vi "Dashboard Main_Fixed_1280x768.vi"() -> ()   [LabVIEW 2023]
uses:
  <vilib>/event_ctls.llb/eventvkey.ctl
  <vilib>/Rock Robotics/Network Tables/NT Read Numeric Array.vi
  <vilib>/Rock Robotics/Network Tables/NT Read Boolean.vi
  <vilib>/Rock Robotics/WPI/Dashboard/WPI_DashboardLogging Global.vi
panel:
  in  "Camera Settings Right":T1={"Frame Rate"=30, "Compression"=30, "Size"=1, "DB Camera Config"=FALSE} {"Frame Rate" scale=1.0..30.0; "Compression" scale=100.0..-1.0; "Size" items=["640x480", "320x240", "160x120"]}
  in  "Camera Name Right":string(combo)="No Camera Selection"
  out "Camera Perf":string
  in  "Camera Settings":T1={"Frame Rate"=30, "Compression"=30, "Size"=1, "DB Camera Config"=FALSE} {"Frame Rate" scale=1.0..30.0; "Compression" scale=100.0..-1.0; "Size" items=["640x480", "320x240", "160x120"]}
  in  "TCP":refnum<k5>
  in  "Rec Mode":enum32{"Stop", "Record", "Playback"}(radio)
  out "Robot IP":string
  out "Image Message":string="Timeout in Camera Communications"
  in  "Dashboard Tab":T2(tab)
  in  "Select Auto":string(combo)="Select Autonomous ..."
  out "NT Connection":bool
  out "MotorChart R":cluster{"Numeric":dbl, "Numeric":dbl}(graph)
  out "MotorChart L":cluster{"Numeric":dbl, "Numeric":dbl}(graph)
  out "MotorSliders R":cluster{"MotorSlide1":dbl, "MotorSlide2":dbl} {"MotorSlide2" scale=-1.0..1.0 scale format="%#_2e"; "MotorSlide1" scale=-1.0..1.0 scale format="%#_2e"}
  out "MotorSliders L":cluster{"MotorSlide1":dbl, "MotorSlide2":dbl} {"MotorSlide2" scale=-1.0..1.0 scale format="%#_2e"; "MotorSlide1" scale=-1.0..1.0 scale format="%#_2e"}
  out "Gyro":dbl(knob) scale=0.0..360.0
  out "JS1 Z":dbl(slide) scale=-1.0..1.0 scale format="%#_2e"
  out "JS1 Graph":cluster{"X":dbl, "Y":dbl}[](graph)
  out "JS1 Buttons":T3
  out "JS2 Z":dbl(slide) scale=-1.0..1.0 scale format="%#_2e"
  out "JS2 Graph":cluster{"X":dbl, "Y":dbl}[](graph)
  out "JS2 Buttons":T3
  out "Mode":T4(ring)=enum."Auto Disabled"
  out "Right Camera Perf":cluster{"Bandwidth (Mbps)":dbl, "FPS":dbl}
  out "Camera Image Right":T5(plugin-control)
  out "State":string
  out "Misaligned":bool
  out "Have Note":bool
  out "Box Ready":bool
  out "Arm on Target":bool
  out "Velocity Deg/Sec":dbl format="%11.1f"
  out "CO":dbl format="%11.2f"
  out "PV Deg":dbl format="%11.1f"
  out "SP Deg":dbl format="%11.1f"
  out "Lower Limit Switch":bool
  out "Arm Chart":T6(graph)
  out "Amp":bool
  out "Arm Blocked":bool
  out "Position":dbl
  out "Demand":dbl
  out "Error":dbl
  out "On Target":bool
  out "Floor":bool
  out "Shoot":bool
  out "Upright":bool
  out "Source":bool
  out "Right Vel":dbl format="%11.1f"
  out "Left Vel":dbl format="%11.1f"
  out "Right On Targ":bool
  out "Left On Targ":bool
  out "Right Upper (Virtual) Limit":bool
  out "Left Upper (Virtual) Limit":bool
  out "Right Low Limit":bool
  out "Right Co":dbl format="%11.2f"
  out "Right PV":dbl format="%11.1f"
  out "Left Co":dbl format="%11.2f"
  out "Left PV":dbl format="%11.1f"
  out "SP Inches":dbl format="%11.1f"
  out "Left Low Limit":bool
  out "Climb Chart":T7(graph)
  out "Left Pos":dbl
  out "Right Pos":dbl
  out "Dmd 2":dbl
  out "Right\nPosition":u8(slide) scale=0.0..100.0
  out "Left\nPosition":u8(slide) scale=0.0..100.0
  out "Dmd":u8(slide) scale=0.0..100.0
  out "Climb Blocked":bool
  out "Selected":string
  out "Step":string
  out "Error Dist":dbl
  in  "Test Slider":dbl(slide) scale=0.0..100.0 scale format="%#_3g"
  in  "On/Off":bool caption="Solenoid"
  in  "Test Name":u16(ring) items=["Select the test to run..."]
  in  "Test Tree":string(tree)
  in  "Motor":cluster{"Value":dbl, "Enable":bool} {"Value" scale=-1.0..1.0 scale format="%#_3g"}
  out "Progress":T8 {"Test Progress" scale=0.0..100.0}
  in  "Rev/Fwd":cluster{"Forward":bool, "Reverse":bool}
  in  "Test Ring":u16(ring) items=["Monochrome", "Color"]
  in  "CheckList":i32(listbox)
  out "Tree":string(tree)
  out "Camera Image":T5(plugin-control)
  out "Background":bool
  in  "Camera Name":string(combo)="No Camera Selection"
  # "HW"
  # "HW"
  # "Joysticks"
  # "Drive Motors"
  # "Front"
  # "Right"
  # "Left"
  # "Back"
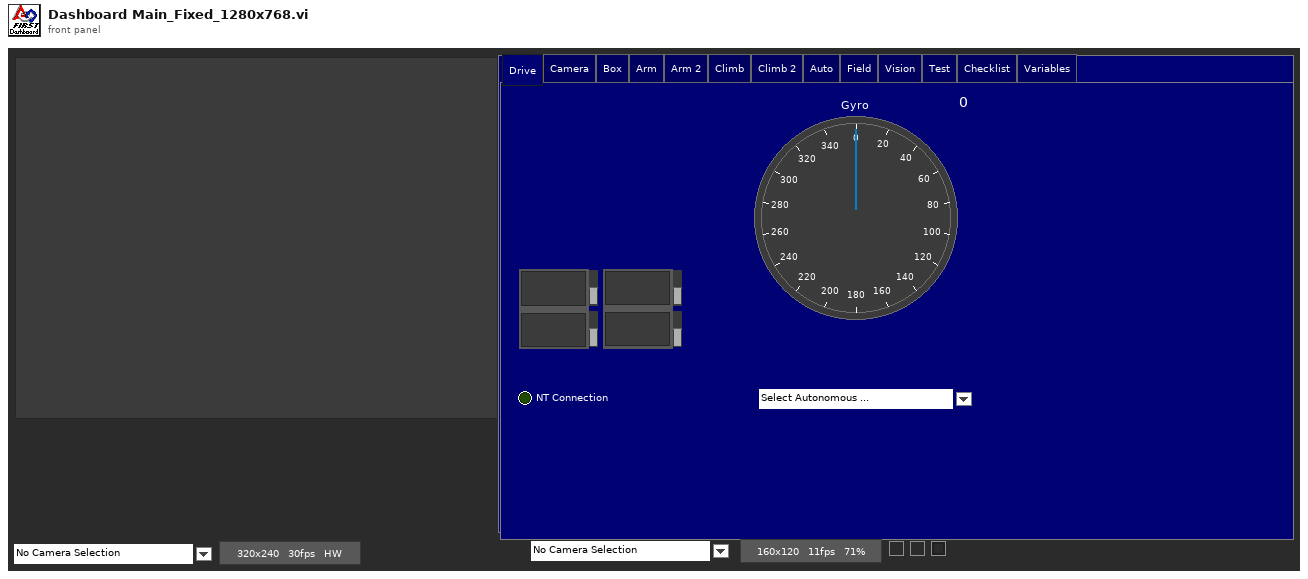
[diagram p1: front panel]
types:
  T1 = cluster{"Frame Rate":i32, "Compression":i32, "Size":u16, "DB Camera Config":bool}
  T2 = enum32{"Drive", "Camera", "Box", "Arm", "Arm 2", "Climb", "Climb 2", "Auto", "Field", "Vision", "Test", "Checklist", "Variables"}
  T3 = cluster{bool, bool, bool, bool, bool, bool, bool, bool, bool, bool, bool, bool}
  T4 = enum8{"Tele-Op Disabled", "Tele-Op Enabled", "Auto Disabled", "Auto Enabled", "Test Disabled", "Test Enabled", "Disconnected", "No Code", "E-Stop"}
  T5 = typedef "IMAQ Image.ctl" = refnum<image>
  T6 = cluster{"value":dbl, "value":dbl, "value":dbl, "value":dbl}
  T7 = cluster{"value":dbl, "value":dbl, "value":dbl, "value":dbl, "value":dbl}
  T8 = cluster{"Test Progress":u8, "Test Progress Text":string}
  T9 = cluster{"Save Path":path, "Interval (s)":dbl, "Keep":i32}
  T10 = enum32{"Drive", "Camera", "Basic", "Custom", "Test", "Commands", "Checklist", "Variables"}
  T11 = typedef "Image Type" = u32
  T12 = cluster{"Error Strings":string, "Disable Counts":cluster{u16, u16}, "Rail Faults":cluster{u16, u16, u16}, "Robot IP":string, "DB Mode":u8, "Event Info":cluster{"Name":string, "Type":u8, "Number":u16, "Replay":u8}}
  T13 = cluster{"Storage":cluster{"Disk Free":u64, "RAM Block":u32, "RAM free":u32}, "CPU Utilization":cluster{"CPU % ISR":sgl, "CPU % Time Crit":sgl, "CPU % Timed Str":sgl, "CPU % High":sgl, "CPU % Above":sgl, "CPU % Normal":sgl, "CPU % Low":sgl}, "CAN":cluster{"% Bus Utilization":sgl, "Bus Off Cnt":u32, "TX_FIFO Full Cnt":u32, "Receive Error Cnt":u8, "Transmit Error Cnt":u8}, "HID":cluster{"HID Outputs":u32, "Rumble Low":u16, "Rumble High":u16}[]}
  T14 = cluster{"Status bits":cluster{"Test Mode":bool, "Autonomous":bool, "Enabled":bool, "Code Start":bool, "Brownout":bool, "Reserved 2":bool, "Reserved 3":bool, "E-Stop":bool}, "Code Trace":cluster{"Disabled":bool, "TeleOp":bool, "Auto":bool, "Test":bool}, "Controller Type":enum16{"unknown", "cRIO", "roboRio"}, "Code?":enum16{"unknown", "noCode", "code"}, "Battery V":dbl}
  T15 = cluster{"Control Bits":cluster{"TestMode":bool, "Autonomous":bool, "Enabled":bool, "FMS Present":bool, bool, bool, bool, "E-Stop":bool}, "Team Station ":u8, "Countdown":sgl, "Joystick Values":cluster{"Axes":dbl[], "Buttons":bool[], "POVs":i16[]}[]}
  T16 = cluster{"Axes":dbl[], "Buttons":bool[], "POVs":i16[]}[]
  T17 = cluster{"Axes":dbl[], "Buttons":bool[], "POVs":i16[]}
  T18 = cluster{"Buttons[0]":bool, "Buttons[1]":bool, "Buttons[2]":bool, "Buttons[3]":bool, "Buttons[4]":bool, "Buttons[5]":bool, "Buttons[6]":bool, "Buttons[7]":bool, "Buttons[8]":bool, "Buttons[9]":bool, "Buttons[10]":bool, "Buttons[11]":bool}
  T19 = cluster{"Camera Image":refnum<vi>, "Dashboard Tab":refnum<vi>, "Background":refnum<vi>, "Rec Mode":refnum<vi>, "Test Slider":refnum<vi>, "On/Off ":refnum<vi>, "Test Ring":refnum<vi>, "Rev/Fwd":refnum<vi>, "Test Name":refnum<vi>, "Motor":refnum<vi>, "Progress":refnum<vi>, "CheckList":refnum<vi>, "Tree":refnum<vi>, "Test Tree":refnum<vi>, "Camera Settings":refnum<vi>, "Camera Name":refnum<vi>, "Camera Perf":refnum<vi>, "Camera Settings Right":refnum<vi>, "Camera Name Right":refnum<vi>, "Camera Image Right":refnum<vi>}
  T20 = cluster{"Global Rectangle":i32[], "Contours":cluster{"Contour Type":u32, "ROI Type":u32, "Points":i32[]}[]}
  T21 = cluster{"Camera Name":string, string, "Saved DB Images Info":cluster{"Save Path":path, "Interval (s)":dbl, "Keep":i32}}
  T22 = cluster{"Camera Name Right":string, string, "Saved DB Images Info":cluster{"Save Path":path, "Interval (s)":dbl, "Keep":i32}}
  T23 = cluster{"Operation":enum16{"Update", "Clear"}, "Color Box":u32}[]
  T24 = typedef "eventvkey.ctl" = enum16{"ASCII", "Enter", "Return", "Shift", "Ctrl", "Alt", "Cmd", "Opt", "Caps", "NumLock", "Clear", "Break", "Up", "Down", "Left", "Right", "Insert", "Delete", "Home", "End", "PageUp", "PageDown", "Escape", "Help", "Pause", "ScrollLock", "F1", "F2", "F3", "F4", "F5", "F6", "F7", "F8", "F9", "F10", "F11", "F12", "F13", "F14", "F15", "F16", "F17", "F18", "F19", "F20", "F21", "F22", "F23", "F24", "Play", "VolumeUp", "VolumeDown", "Mute", "Two Byte Char"}
  T25 = cluster{"Image Size":bool, "Image Type":bool, "Pixel Value":bool, "ROI Information":bool, "Zoom Factor":bool}
  T26 = cluster{"Operation":enum16{"Update", "Clear"}, "Color Box":u32}
  T27 = cluster{"Shift":bool, "Ctrl":bool, "Alt":bool, "Cmd":bool, "Opt":bool}
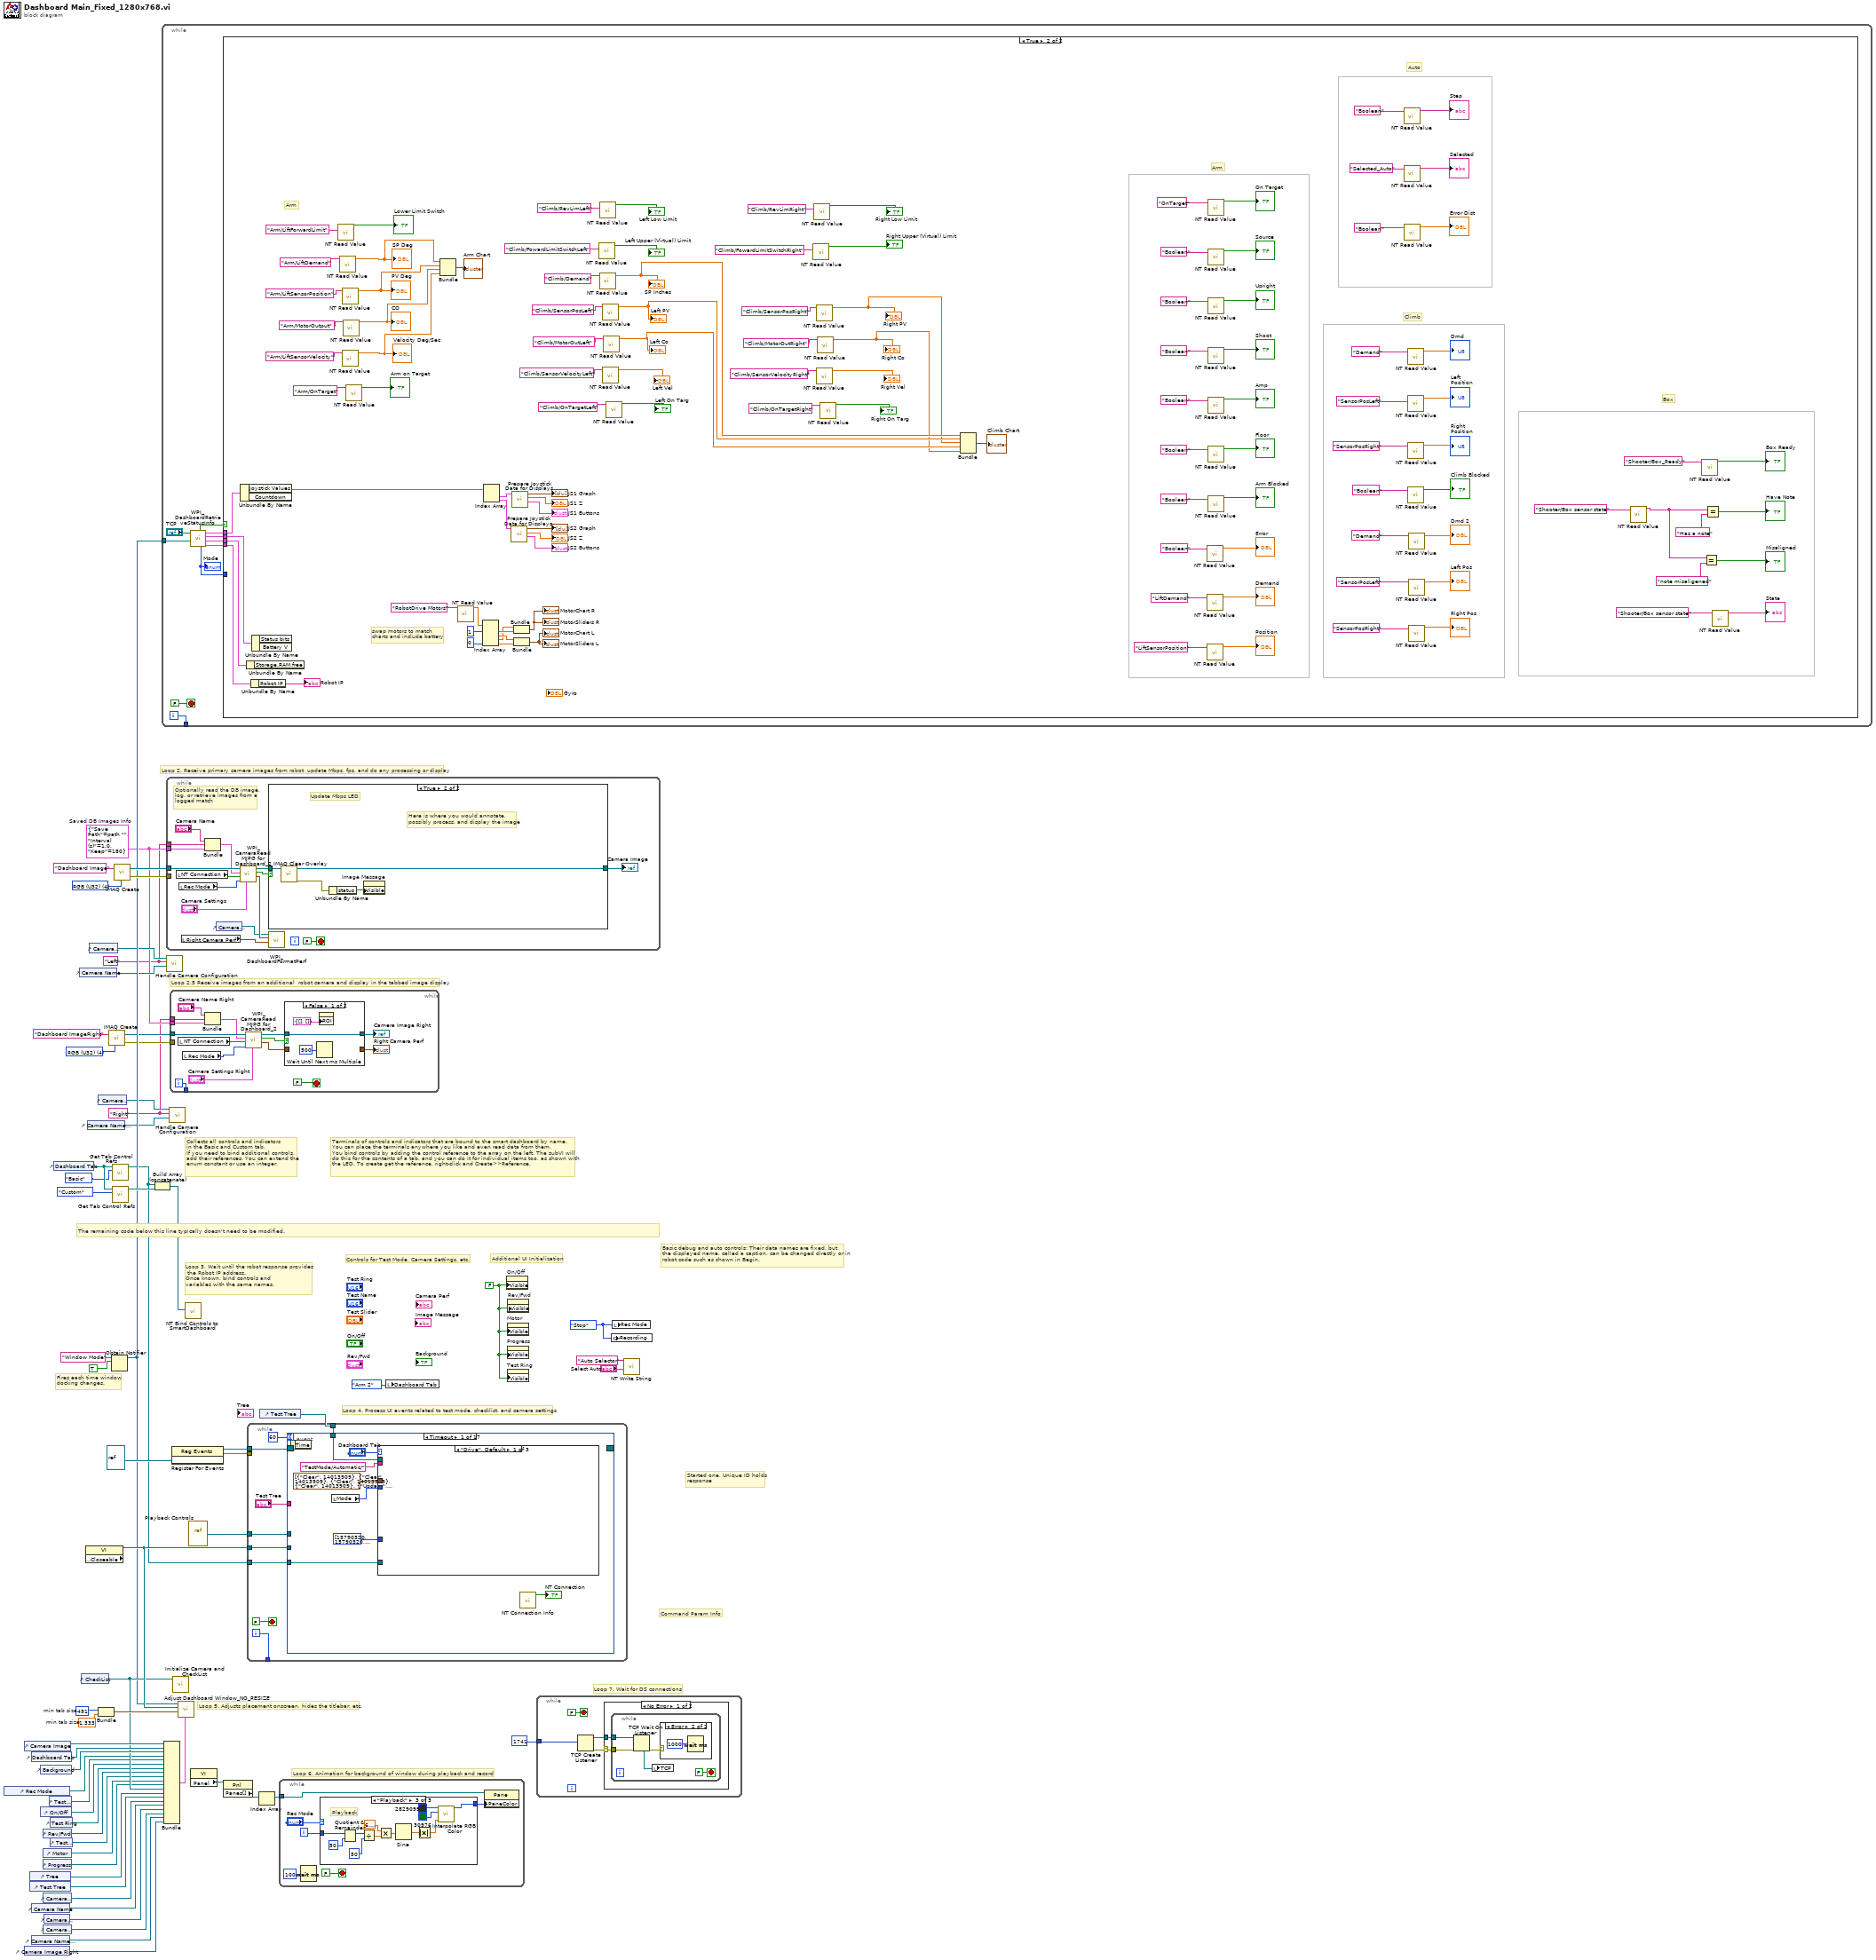
[diagram p0: block diagram]
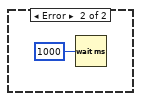
[diagram p4: hidden frame]
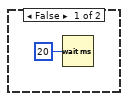
[diagram p5: hidden frame]
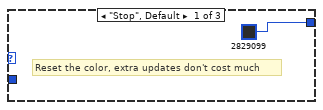
[diagram p6: hidden frame]
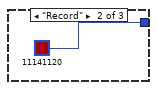
[diagram p7: hidden frame]
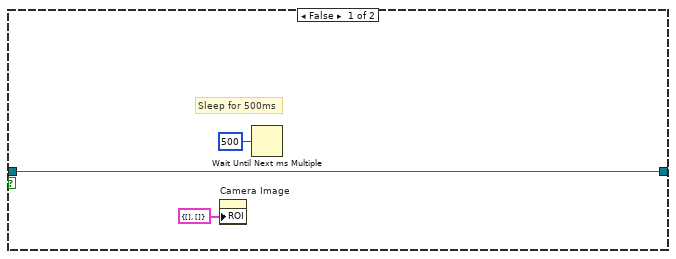
[diagram p8: hidden frame]
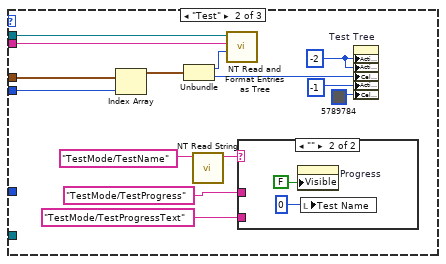
[diagram p9: hidden frame]
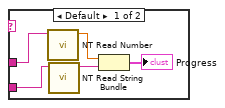
[diagram p10: hidden frame]
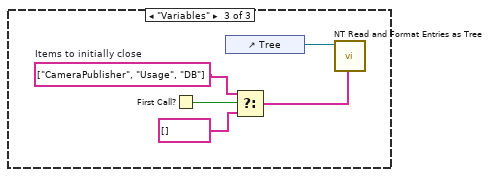
[diagram p11: hidden frame]
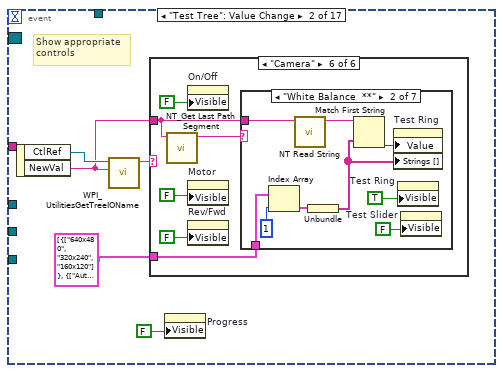
[diagram p12: hidden frame]
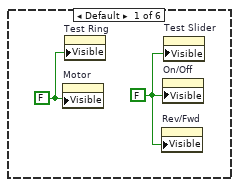
[diagram p13: hidden frame]
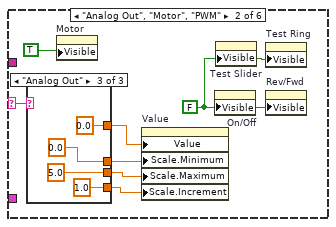
[diagram p14: hidden frame]
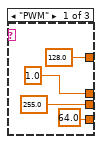
[diagram p15: hidden frame]
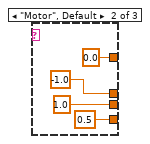
[diagram p16: hidden frame]
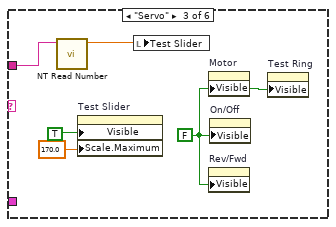
[diagram p17: hidden frame]
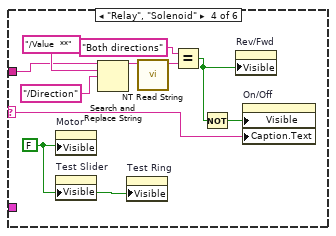
[diagram p18: hidden frame]
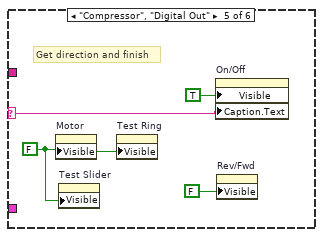
[diagram p19: hidden frame]
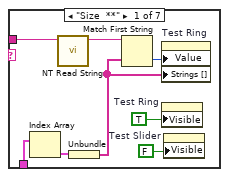
[diagram p20: hidden frame]
diagram:
  w4 = T9 {"Save Path"=path "", "Interval (s)"=1.0, "Keep"=180}  # Saved DB Images Info
  w3 = "Right"
  w2 = "Left"
  w14 = T11 4 items=["Grayscale (U8)", "Grayscale (I16)", "Grayscale (SGL)", "Complex (CSG)", "RGB (U32)", "HSL (U32)", "RGB (U64)"] ("Image Type")
  w42 = 491  # min tab size
  w41 = 1.333  # min tab size
  w49 = enum32{"Stop", "Record", "Playback"}."Stop" ("Rec Mode")
  w26 = FALSE ("Visible")
  w63 = T11 4 items=["Grayscale (U8)", "Grayscale (I16)", "Grayscale (SGL)", "Complex (CSG)", "RGB (U32)", "HSL (U32)", "RGB (U64)"] ("Image Type")
  # "Loop 2.5 Receive images from an additional  robot camera and display in the tabbed image display"
  # "Command Param Info"
  # "Started one, Unique ID holds\nresponse"
  # "Loop 7. Wait for DS connections"
  # "Basic debug and auto controls: Their data names are fixed, but\nthe displayed name, called a caption, can be changed directly or in\nrobot code such as shown in Begin."
  # "Controls for Test Mode, Camera Settings, etc."
  # "Additional UI Initialization"
  # "Loop 6. Animation for background of window during playback and record"
  # "Fires each time window\ndocking changes."
  # "Collects all controls and indicators\nin the Basic and Custom tab.\nIf you need to bind additional controls,\nadd their references. You can extend the\nenum constant or use an integer."
  # "The remaining code below this line typically doesn't need to be modified."
  # "Loop 4. Process UI events related to test mode, checklist, and camera settings"
  # "Terminals of controls and indicators that are bound to the smart dashboard by name.\nYou can place the terminals anywhere you like and even read data from them.\nYou bind controls by adding the control reference to the array on the left. The subVI will\ndo this for the contents of a tab, and you can do it for individual items too, as shown with\nthe LED. To create get the reference, right-click and Create>>Reference."
  # "Loop 3. Wait until the robot response provides\n the Robot IP address.\nOnce known, bind controls and\nvariables with the same names."
  # "Loop 5. Adjusts placement onscreen, hides the titlebar, etc."
  # "Loop 2. Receive primary camera images from robot, update Mbps, fps, and do any processing or display"
  n1 = control-ref of="Rec Mode"() -> (w32:refnum<vi>)
  n2 = control-ref of="Camera Image Right"() -> (w7:refnum<vi>)
  n3 = control-ref of="Camera Image"() -> (w44:refnum<vi>)
  n4 = control-ref of="Tree"() -> (w36:refnum<vi>)
  n5 = control-ref of="Test Tree"() -> (w35:refnum<vi>)
  n6 = control-ref of="Dashboard Tab"() -> (w43:refnum<vi>)
  n7 = control-ref of="Camera Name"() -> (w20:refnum<vi>)
  n8 = control-ref of="Camera Name Right"() -> (w8:refnum<vi>)
  n9 = control-ref of="Background"() -> (w39:refnum<vi>)
  n10 = control-ref of="On/Off"() -> (w30:refnum<vi>)
  n11 = control-ref of="Progress"() -> (w27:refnum<vi>)
  n12 = control-ref of="Camera Settings"() -> (w21:refnum<vi>)
  n13 = control-ref of="Camera Settings Right"() -> (w9:refnum<vi>)
  n14 = control-ref of="Rev/Fwd"() -> (w28:refnum<vi>)
  n15 = control-ref of="Motor"() -> (w33:refnum<vi>)
  n16 = control-ref of="Camera Perf"() -> (w19:refnum<vi>)
  n17 = control-ref of="Test Slider"() -> (w31:refnum<vi>)
  n18 = control-ref of="Test Ring"() -> (w29:refnum<vi>)
  n19 = control-ref of="Test Name"() -> (w34:refnum<vi>)
  n20 = control-ref of="Dashboard Tab"() -> (w47:refnum<vi>)
  n21 = control-ref of="Camera Name"() -> (w22:refnum<vi>)
  n22 = control-ref of="CheckList"() -> (w37:refnum<vi>)
  n23 = property class="VI" props=["Front Panel.Closeable"]() -> (reference out=w48:refnum<vi>)  [unwired: 2 in, 2 out]
  n24 = control-ref of="Camera Name Right"() -> (w10:refnum<vi>)
  n25 = control-ref of="Camera Settings"() -> (w23:refnum<vi>)
  n26 = control-ref of="Camera Settings Right"() -> (w11:refnum<vi>)
  n27 = Bundle("min tab size"=w42, "min tab size"=w41) -> (w40:cluster{"min tab size":i32, "min tab size":dbl})  [unwired: 1 in]
  n28 = call "IMAQ Create"("Image Name"="Dashboard ImageRight", "Image Type"=w14) -> ("New Image"=w13:T5, "error out"=w12:errorcluster)  [unwired: 2 in, 1 out]
  n29 = Obtain Notifier(name (unnamed)="Window Mode", notification data type=TRUE) -> (notifier out=w25:refnum<notifier>)  [unwired: 2 in, 2 out]
  n30 = call <vilib>:"Get Tab Control Refs.vi"("Page Index"=T10."Basic" ("Dashboard Tab"), "TabControl in"=w47) -> ("ControlsOnPage"=w18:refnum<vi>[])  [unwired: 9 in]
  n31 = call <vilib>:"Get Tab Control Refs.vi"("Page Index"=T10."Custom" ("Dashboard Tab"), "TabControl in"=w47) -> ("ControlsOnPage"=w46:refnum<vi>[])  [unwired: 9 in]
  n32 = call "IMAQ Create"("Image Name"="Dashboard Image", "Image Type"=w63) -> ("New Image"=w61:T5, "error out"=w60:errorcluster)  [unwired: 2 in, 1 out]
  n33 = Build Array (concatenate)(w18, w46) -> (w45:refnum<vi>[])
  n34 = while {
    tunnel: [w72] -> _
    tunnel: w25 -> [w64]
    i -> [w72]
    stop <- FALSE stop-if-true
    n35 = call <vilib>:"WPI_DashboardRetrieveStatusInfo.vi"("Window Mode Notifier"=w64, "TCP Cnx"="TCP") -> ("Power and Errors"=w67:T12, "Robot Metrics"=w70:T13, "Status Info"=w71:T14, "Control Info"=w68:T15, "Robot Mode"=w66:T4, "Process?"=w69:bool)  [unwired: 4 in]
    "Mode" <- w66
    n36 = case shown="True" w69 {
      tunnel: w71 -> [_ w188]
      tunnel: w70 -> [_ w187]
      tunnel: w68 -> [_ w186]
      tunnel: w67 -> [_ w185]
      tunnel: w66 -> [_ _]
      frame False {
        n37 = Wait (ms)(milliseconds to wait=u32 20) -> ()  [unwired: 1 out]
      }
      frame True {
        # "Auto"
        # "Climb"
        # "Arm"
        # "Box"
        # "Arm"
        # "swap motors to match\ncharts and include battery"
        n38 = Unbundle By Name(w186) -> ("Joystick Values"=w176:T16)  [unwired: 1 out]
        n39 = Unbundle By Name(w187) -> ()  [unwired: 1 out]
        n40 = Unbundle By Name(w185) -> ("Robot IP"=→"Robot IP":string)
        n41 = Unbundle By Name(w188) -> ()  [unwired: 2 out]
        n42 = call-poly <vilib>:"NT Read Value.vi"("name"="Arm/LiftForwardLimit") -> ("value"=→"Lower Limit Switch":bool)  [unwired: 8 in, 2 out]
        n43 = call-poly <vilib>:"NT Read Value.vi"("name"="Arm/LiftDemand") -> ("value"=w156:dbl)  [unwired: 8 in, 2 out]
        "SP Deg" <- w156
        n44 = call-poly <vilib>:"NT Read Value.vi"("name"="Arm/LiftSensorPosition") -> ("value"=w155:dbl)  [unwired: 8 in, 2 out]
        "PV Deg" <- w155
        n45 = call-poly <vilib>:"NT Read Value.vi"("name"="Arm/LiftSensorVelocity") -> ("value"=w153:dbl)  [unwired: 8 in, 2 out]
        "Velocity Deg/Sec" <- w153
        n46 = call-poly <vilib>:"NT Read Value.vi"("name"="Arm/MotorOutput") -> ("value"=w154:dbl)  [unwired: 8 in, 2 out]
        "CO" <- w154
        n47 = call-poly <vilib>:"NT Read Value.vi"("name"="Arm/OnTarget") -> ("value"=→"Arm on Target":bool)  [unwired: 8 in, 2 out]
        n48 = Bundle("value"=w156, "value"=w155, "value"=w154, "value"=w153) -> (→"Arm Chart":T6)  [unwired: 1 in]
        n49 = call-poly <vilib>:"NT Read Value.vi"("name"="RobotDrive Motors" ("Name")) -> ("value"=w166:dbl[])  [unwired: 8 in, 2 out]
        n50 = Index Array(array=w166, index #1=1, index #4=0) -> (element #1=w180:dbl, element #2=w181:dbl, element #3=w179:dbl, element #4=w184:dbl)  [unwired: 2 in]
        n51 = Index Array(array=w176) -> (element #1=w175:T17, element #2=w171:T17)  [unwired: 2 in]
        n52 = call "Prepare Joystick Data for Displays.vi"("Joystick Values"=w171) -> ("Buttons"=→"JS2 Buttons":T18, "Z Axis"=→"JS2 Z":dbl, "Cartesian Data"=→"JS2 Graph":cluster{"X axis":dbl, "X axis":dbl}[])  [unwired: 8 in]
        n53 = call "Prepare Joystick Data for Displays.vi"("Joystick Values"=w175) -> ("Buttons"=→"JS1 Buttons":T18, "Z Axis"=→"JS1 Z":dbl, "Cartesian Data"=→"JS1 Graph":cluster{"X axis":dbl, "X axis":dbl}[])  [unwired: 8 in]
        n54 = Bundle("Numeric"=w179, "Numeric"=w180) -> (→"MotorChart R" →"MotorSliders R":cluster{"Numeric":dbl, "Numeric":dbl})  [unwired: 1 in]
        n55 = Bundle("Numeric"=w181, "Numeric"=w184) -> (→"MotorChart L" →"MotorSliders L":cluster{"Numeric":dbl, "Numeric":dbl})  [unwired: 1 in]
        n56 = call-poly <vilib>:"NT Read Value.vi"("name"="Climb/FowardLimitSwitchLeft") -> ("value"=→"Left Upper (Virtual) Limit":bool)  [unwired: 8 in, 2 out]
        n57 = call-poly <vilib>:"NT Read Value.vi"("name"="Climb/Demand") -> ("value"=w129:dbl)  [unwired: 8 in, 2 out]
        "SP Inches" <- w129
        n58 = call-poly <vilib>:"NT Read Value.vi"("name"="Climb/RevLimLeft") -> ("value"=→"Left Low Limit":bool)  [unwired: 8 in, 2 out]
        n59 = call-poly <vilib>:"NT Read Value.vi"("name"="Climb/SensorPosLeft") -> ("value"=w128:dbl)  [unwired: 8 in, 2 out]
        "Left PV" <- w128
        n60 = call-poly <vilib>:"NT Read Value.vi"("name"="Climb/SensorVelocityLeft") -> ("value"=→"Left Vel":dbl)  [unwired: 8 in, 2 out]
        n61 = call-poly <vilib>:"NT Read Value.vi"("name"="Climb/MotorOutLeft") -> ("value"=w126:dbl)  [unwired: 8 in, 2 out]
        "Left Co" <- w126
        n62 = call-poly <vilib>:"NT Read Value.vi"("name"="Climb/OnTargetLeft") -> ("value"=→"Left On Targ":bool)  [unwired: 8 in, 2 out]
        n63 = call-poly <vilib>:"NT Read Value.vi"("name"="Climb/FowardLimitSwitchRight") -> ("value"=→"Right Upper (Virtual) Limit":bool)  [unwired: 8 in, 2 out]
        n64 = call-poly <vilib>:"NT Read Value.vi"("name"="Climb/RevLimRight") -> ("value"=→"Right Low Limit":bool)  [unwired: 8 in, 2 out]
        n65 = call-poly <vilib>:"NT Read Value.vi"("name"="Climb/SensorPosRight") -> ("value"=w127:dbl)  [unwired: 8 in, 2 out]
        "Right PV" <- w127
        n66 = call-poly <vilib>:"NT Read Value.vi"("name"="Climb/SensorVelocityRight") -> ("value"=→"Right Vel":dbl)  [unwired: 8 in, 2 out]
        n67 = call-poly <vilib>:"NT Read Value.vi"("name"="Climb/MotorOutRight") -> ("value"=w125:dbl)  [unwired: 8 in, 2 out]
        "Right Co" <- w125
        n68 = call-poly <vilib>:"NT Read Value.vi"("name"="Climb/OnTargetRight") -> ("value"=→"Right On Targ":bool)  [unwired: 8 in, 2 out]
        n69 = Bundle("value"=w129, "value"=w128, "value"=w127, "value"=w126, "value"=w125) -> (→"Climb Chart":T7)  [unwired: 1 in]
        n70 = call-poly <vilib>:"NT Read Value.vi"("name"="Boolean") -> ("value"=→"Error":dbl)  [unwired: 8 in, 2 out]
        n71 = call-poly <vilib>:"NT Read Value.vi"("name"="LiftDemand") -> ("value"=→"Demand":dbl)  [unwired: 8 in, 2 out]
        n72 = call-poly <vilib>:"NT Read Value.vi"("name"="LiftSensorPosition") -> ("value"=→"Position":dbl)  [unwired: 8 in, 2 out]
        n73 = call-poly <vilib>:"NT Read Value.vi"("name"="OnTarget") -> ("value"=→"On Target":bool)  [unwired: 8 in, 2 out]
        n74 = call-poly <vilib>:"NT Read Value.vi"("name"="Boolean") -> ("value"=→"Source":bool)  [unwired: 8 in, 2 out]
        n75 = call-poly <vilib>:"NT Read Value.vi"("name"="Boolean") -> ("value"=→"Upright":bool)  [unwired: 8 in, 2 out]
        n76 = call-poly <vilib>:"NT Read Value.vi"("name"="Boolean") -> ("value"=→"Shoot":bool)  [unwired: 8 in, 2 out]
        n77 = call-poly <vilib>:"NT Read Value.vi"("name"="Boolean") -> ("value"=→"Amp":bool)  [unwired: 8 in, 2 out]
        n78 = call-poly <vilib>:"NT Read Value.vi"("name"="Boolean") -> ("value"=→"Floor":bool)  [unwired: 8 in, 2 out]
        n79 = call-poly <vilib>:"NT Read Value.vi"("name"="Boolean") -> ("value"=→"Arm Blocked":bool)  [unwired: 8 in, 2 out]
        n80 = call-poly <vilib>:"NT Read Value.vi"("name"="Boolean") -> ("value"=→"Step":string)  [unwired: 8 in, 2 out]
        n81 = call-poly <vilib>:"NT Read Value.vi"("name"="Selected_Auto") -> ("value"=→"Selected":string)  [unwired: 8 in, 2 out]
        n82 = call-poly <vilib>:"NT Read Value.vi"("name"="Boolean") -> ("value"=→"Error Dist":dbl)  [unwired: 8 in, 2 out]
        n83 = call-poly <vilib>:"NT Read Value.vi"("name"="Demand") -> ("value"=→"Dmd":dbl)  [unwired: 8 in, 2 out]
        n84 = call-poly <vilib>:"NT Read Value.vi"("name"="SensorPosLeft") -> ("value"=→"Left\nPosition":dbl)  [unwired: 8 in, 2 out]
        n85 = call-poly <vilib>:"NT Read Value.vi"("name"="SensorPosRight") -> ("value"=→"Right\nPosition":dbl)  [unwired: 8 in, 2 out]
        n86 = call-poly <vilib>:"NT Read Value.vi"("name"="Boolean") -> ("value"=→"Climb Blocked":bool)  [unwired: 8 in, 2 out]
        n87 = call-poly <vilib>:"NT Read Value.vi"("name"="Demand") -> ("value"=→"Dmd 2":dbl)  [unwired: 8 in, 2 out]
        n88 = call-poly <vilib>:"NT Read Value.vi"("name"="SensorPosLeft") -> ("value"=→"Left Pos":dbl)  [unwired: 8 in, 2 out]
        n89 = call-poly <vilib>:"NT Read Value.vi"("name"="SensorPosRight") -> ("value"=→"Right Pos":dbl)  [unwired: 8 in, 2 out]
        n90 = call-poly <vilib>:"NT Read Value.vi"("name"="Shooter/Box sensor state") -> ("value"=w77:string)  [unwired: 8 in, 2 out]
        n91 = call-poly <vilib>:"NT Read Value.vi"("name"="Shooter/Box_Ready") -> ("value"=→"Box Ready":bool)  [unwired: 8 in, 2 out]
        n92 = Equal?(x=w77, y="note misaligened") -> (x = y?=→"Misaligned":bool)
        n93 = Equal?(x=w77, y="Has a note") -> (x = y?=→"Have Note":bool)
        n94 = call-poly <vilib>:"NT Read Value.vi"("name"="Shooter/Box sensor state") -> ("value"=→"State":string)  [unwired: 8 in, 2 out]
      }
    }
  }
  n95 = Bundle("Camera Image"=w44, "Dashboard Tab"=w43, "Background"=w39, "Rec Mode"=w32, "Test Slider"=w31, "On/Off"=w30, "Test Ring"=w29, "Rev/Fwd"=w28, "Test Name"=w34, "Motor"=w33, "Progress"=w27, "CheckList"=w37, "Tree"=w36, "Test Tree"=w35, "Camera Settings"=w21, "Camera Name"=w20, "Camera Perf"=w19, "Camera Settings Right"=w9, "Camera Name Right"=w8, "Camera Image Right"=w7) -> (w38:T19)  [unwired: 1 in]
  n96 = call "Handle Camera Configuration.vi"("CameraNameRef"=w22, "Display Name"=w2, "ClusterRef"=w23) -> ()  [unwired: 9 in]
  n97 = while {
    tunnel: w61 -> [w202]
    tunnel: w60 -> [_]
    tunnel: w4 -> [w195]
    tunnel: w2 -> [w192]
    stop <- FALSE stop-if-true
    # "Optionally read the DB image,\nlog, or retrieve images from a\nlogged match"
    n98 = local read "NT Connection"() -> (w196:bool)
    n99 = local read "Rec Mode"() -> (w199:enum32{"Stop", "Record", "Playback"})
    n100 = local read "Right Camera Perf"() -> (w190:cluster{"Bandwidth (Mbps)":dbl, "FPS":dbl})
    n101 = Bundle("Camera Name"="Camera Name", w192, "Saved DB Images Info"=w195) -> (w194:T21)  [unwired: 1 in]
    n102 = control-ref of="Camera Perf"() -> (w189:refnum<vi>)
    n103 = call <vilib>:"WPI_CameraRead MJPG for Dashboard_2.vi"("Camera Settings"="Camera Settings", "Rec Mode"=w199, "NT Connection"=w196, "Capture Info"=w194, "Image in"=w202) -> ("perf info"=w191:cluster{"Bandwidth (Mbps)":dbl, "fps":dbl}, "Active"=w200:bool, "Image\\ out"=w201:T5)  [unwired: 4 in]
    n104 = case shown="True" w200 {
      tunnel: w201 -> [w205 w208]
      tunnel: [w205 w207] -> w197
      frame False {
        # "Sleep for 500ms"
        n105 = property on="Camera Image" class="ImageControl"("ROI"=T20 {"Global Rectangle"=[], "Contours"=[]}) -> ()  [unwired: 2 in, 2 out]
        n106 = Wait Until Next ms Multiple(millisecond multiple=u32 500) -> ()  [unwired: 1 out]
      }
      frame True {
        # "Here is where you would annotate,\npossibly process, and display the image"
        # "Update Mbps LED"
        n107 = call "IMAQ Clear Overlay"("Image"=w208) -> ("error out"=w209:errorcluster, "Image Out"=w207:T5)  [unwired: 2 in, 7 out]
        n108 = Unbundle By Name(w209) -> ("status"=w210:bool)
        n109 = property on="Image Message" class="Str"("Visible"=w210) -> ()  [unwired: 2 in, 2 out]
      }
    }
    "Camera Image" <- w197
    n110 = call <vilib>:"WPI_DashboardFormatPerf.vi"("Right Camera Perf"=w190, "Performance"=w191, "String in"=w189) -> ()  [unwired: 9 in]
  }
  n111 = call "Handle Camera Configuration.vi"("CameraNameRef"=w10, "Display Name"=w3, "ClusterRef"=w11) -> ()  [unwired: 9 in]
  n112 = while {
    tunnel: w13 -> [w225]
    tunnel: w12 -> [_]
    tunnel: [w220] -> _
    tunnel: w4 -> [w216]
    tunnel: w3 -> [w213]
    i -> [w220]
    stop <- FALSE stop-if-true
    n113 = local read "NT Connection"() -> (w217:bool)
    n114 = local read "Rec Mode"() -> (w224:enum32{"Stop", "Record", "Playback"})
    n115 = Bundle("Camera Name Right"="Camera Name Right", w213, "Saved DB Images Info"=w216) -> (w215:T22)  [unwired: 1 in]
    n116 = call <vilib>:"WPI_CameraRead MJPG for Dashboard_2.vi"("Camera Settings"="Camera Settings Right", "Rec Mode"=w224, "NT Connection"=w217, "Capture Info"=w215, "Image in"=w225) -> ("perf info"=w211:cluster{"Bandwidth (Mbps)":dbl, "fps":dbl}, "Active"=w219:bool, "Image\\ out"=w222:T5)  [unwired: 4 in]
    n117 = case shown="False" w219 {
      tunnel: w222 -> [w227 w230]
      tunnel: [w227 w230] -> w218
      tunnel: [_ w229] -> w212
      tunnel: w211 -> [_ w229]
      frame False {
        n118 = Wait Until Next ms Multiple(millisecond multiple=u32 500) -> ()  [unwired: 1 out]
        n119 = property on="Camera Image Right" class="ImageControl"("ROI"=T20 {"Global Rectangle"=[], "Contours"=[]}) -> ()  [unwired: 2 in, 2 out]
      }
      frame True {
      }
    }
    "Camera Image Right" <- w218
    "Right Camera Perf" <- w212
  }
  n120 = register-events(refnum<vi> refnum) -> (reference out=w52:refnum<event-registration>, error out=w51:errorcluster)  [unwired: 2 in]
  n121 = call "Initialize Camera and CheckList.vi"("ListBox in"=w37) -> ()  [unwired: 11 in]
  n122 = call "Adjust Dashboard Window_NO_RESIZE.vi"("Sizing Refnums"=w38, "Size Constraints"=w40, "VI"=w48, "WIn Mode"=w25) -> ()  [unwired: 8 in]
  n123 = call <vilib>:"NT Bind Controls to SmartDashboard.vi"("Bound Control Refs"=w45) -> ()  [unwired: 11 in]
  n124 = vi-ref "Playback Controls.vi"() -> (w53:refnum<vi>)
  n125 = property class="VI"() -> ("Panel"=w55:refnum<vi>)  [unwired: 2 in, 2 out]
  n126 = property class="Pnl"(reference=w55) -> ("Panes[]"=w56:refnum<vi>[])  [unwired: 1 in, 2 out]
  n127 = Index Array(array=w56) -> (element=w54:refnum<vi>)  [unwired: 1 in]
  n128 = control-ref of="Test Tree"() -> (w57:refnum<vi>)
  n129 = while {
    tunnel: [w236] -> _
    tunnel: w57 -> [w235]
    tunnel: w53 -> [w234]
    tunnel: w52 -> [w233]
    tunnel: w51 -> [_]
    tunnel: w48 -> [w232]
    tunnel: w18 -> [w231]
    i -> [w236]
    stop <- FALSE stop-if-true
    n130 = event shown="[0] Timeout" {
      selector: w233 -> [_ _ _ _ _ _ _ _ _ _ _ _ _ _ _ _ _]
      dyn-events: [_ _ _ _ _ _ _ _ _ _ _ _ _ w440 _ _ _] -> _
      timeout: u32 60 ("milliseconds to wait") -> [_ _ _ _ _ _ _ _ _ _ _ _ _ _ _ _ _]
      tunnel: w235 -> [w246 _ _ _ _ _ _ _ _ _ _ _ _ _ _ _ _]
      tunnel: "Test Tree" -> [_ _ _ _ _ _ _ _ w413 w420 w421 w424 w431 _ _ _ _]
      tunnel: w234 -> [_ _ _ _ _ _ _ _ _ _ _ _ _ w442 _ w457 _]
      tunnel: w232 -> [_ _ _ _ _ _ _ _ _ _ _ _ _ w438 _ _ _]
      tunnel: w231 -> [w241 _ _ _ _ _ _ _ _ _ _ _ _ _ _ _ _]
      event Timeout {
        n131 = event-data() -> ()  [unwired: 1 in, 1 out]
        n132 = local read "Mode"() -> (w244:T4)
        n133 = case shown="\"Drive\", Default" "Dashboard Tab" {
          tunnel: w246 -> [_ w261 _]
          tunnel: "TestMode/Automatic/" ("Name Pattern") -> [_ w260 _]
          tunnel: T23 [{"Operation"=enum."Clear", "Color Box"=14013909}, {"Operation"=enum."Clear", "Color Box"=14013909}, {"Operation"=enum."Clear", "Color Box"=14013909}, {"Operation"=enum."Clear", "Color Box"=14013909}, {"Operation"=enum."Update", "Color Box"=14013909}, {"Operation"=enum."Update", "Color Box"=16777215}, {"Operation"=enum."Clear", "Color Box"=14013909}, {"Operation"=enum."Clear", "Color Box"=14013909}, {"Operation"=enum."Clear", "Color Box"=14013909}] -> [_ w253 _]
          tunnel: w244 -> [_ w252 _]
          tunnel: u32[] [15790320, 15790320, 15790320, 15790320, 16777215, 16777215, 15790320, 15790320, 15790320] -> [_ _ _]
          tunnel: w241 -> [_ _ _]
          frame "Drive", Default {
          }
          frame "Test" {
            w259 = -2 ("Active Item:Row Number")
            n134 = Index Array(array=w253, index=w252) -> (element=w254:T26)
            n135 = Unbundle(w254) -> ("Operation"=w255:enum16{"Update", "Clear"}, "Color Box"=w256:u32)
            n136 = call <vilib>:"NT Read String.vi"("name"="TestMode/TestName" ("Name")) -> ("value"=w250:string)  [unwired: 8 in, 2 out]
            n137 = call <vilib>:"NT Read and Format Entries as Tree.vi"("Operation"=w255, "Name Pattern"=w260, "Tree Refnum"=w261) -> ()  [unwired: 7 in, 2 out]
            n138 = case shown="\"\"" w250 {
              tunnel: "TestMode/TestProgress" ("Name") -> [w263 _]
              tunnel: "TestMode/TestProgressText" ("Name") -> [w262 _]
              frame Default {
                n139 = call <vilib>:"NT Read Number.vi"("name"=w263) -> ("value"=w264:dbl)  [unwired: 8 in, 2 out]
                n140 = call <vilib>:"NT Read String.vi"("name"=w262) -> ("value"=w265:string)  [unwired: 8 in, 2 out]
                n141 = Bundle("value"=w264, "value"=w265) -> (→"Progress":cluster{"value":dbl, "value":string})  [unwired: 1 in]
              }
              frame "" {
                n142 = property on="Progress" class="Clust (strict)"("Visible"=FALSE) -> ()  [unwired: 2 in, 2 out]
                n143 = local write "Test Name"(u16 0) -> ()
              }
            }
            n144 = property on="Test Tree" class="Tree (strict)"("Active Item Row Number"=w259, "ActiveColNum"=w259, "CellBG"=w256, "Active Item Row Number"=-1 ("Active Item:Row Number"), "CellBG"=u32 5789784 ("Color Box")) -> ()  [unwired: 2 in, 2 out]
          }
          frame "Variables" {
            w271 = string[] ["CameraPublisher", "Usage", "DB"]  # Items to initially close
            n145 = First Call?() -> (First Call?: T/F=w272:bool)
            n146 = control-ref of="Tree"() -> (w273:refnum<vi>)
            n147 = Select(t=w271, s=w272, f=string[] []) -> (s? t:f=w269:string[])
            n148 = call <vilib>:"NT Read and Format Entries as Tree.vi"("Tags to  Close"=w269, "Tree Refnum"=w273) -> ()  [unwired: 8 in, 2 out]
          }
        }
        n149 = call <vilib>:"NT Connection Info.vi"() -> ("Connected"=→"NT Connection":bool)  [unwired: 11 in]
      }
      event "Test Tree": Value Change {
        # "Show appropriate\ncontrols"
        n150 = event-data() -> ("CtlRef"=w277:refnum<vi>, "NewVal"=w275:string)  [unwired: 1 in]
        n151 = call <vilib>:"WPI_UtilitiesGetTreeIOName.vi"("NewVal"=w275, "TreeControl in"=w277) -> ("I/O Name"=w278:string)  [unwired: 9 in]
        n152 = case shown="\"Camera\"" w278 {
          selector: w278 -> [_ w285 _ w307 w316 _]
          tunnel: w275 -> [_ _ w304 w306 _ w323]
          tunnel: cluster{string[]}[] [{["640x480", "320x240", "160x120"]}, {["Auto", "Fixed indoor", "Fixed outdoor 1", "Fixed outdoor 2", "Fixed fluorescent 1", "Fixed fluorescent 2", "Hold current"]}, {["Auto", "Flicker-free 50 Hz", "Flicker-free 60 Hz", "Hold current"]}, {["None", "Prioritize frame rate", "Prioritize image quality"]}, {["Monochrome", "Color"]}] -> [_ _ _ _ _ w322]
          frame Default {
            w280 = FALSE ("Visible")
            w279 = FALSE ("Visible")
            n153 = property on="Motor" class="Clust (strict)"("Visible"=w279) -> ()  [unwired: 2 in, 2 out]
            n154 = property on="Test Ring" class="Ring (strict)"("Visible"=w279) -> ()  [unwired: 2 in, 2 out]
            n155 = property on="Rev/Fwd" class="Clust (strict)"("Visible"=w280) -> ()  [unwired: 2 in, 2 out]
            n156 = property on="On/Off" class="Bool (strict)"("Visible"=w280) -> ()  [unwired: 2 in, 2 out]
            n157 = property on="Test Slider" class="Slide (strict)"("Visible"=w280) -> ()  [unwired: 2 in, 2 out]
          }
          frame "Analog Out", "Motor", "PWM" {
            w286 = FALSE ("Visible")
            n158 = case shown="\"Analog Out\"" w285 {
              tunnel: [1.0 ("Value") -1.0 ("Value") 0.0 ("Value")] -> w284
              tunnel: [255.0 ("Value") 1.0 ("Value") 5.0 ("Value")] -> w283
              tunnel: [128.0 ("Value") 0.0 ("Value") 0.0 ("Value")] -> w282
              tunnel: [64.0 ("Value") 0.5 ("Value") 1.0 ("Value")] -> w281
              frame "PWM" {
              }
              frame "Motor", Default {
              }
              frame "Analog Out" {
              }
            }
            n159 = property on="Motor" class="Clust (strict)"("Visible"=TRUE) -> ()  [unwired: 2 in, 2 out]
            n160 = property on="Value" class="Slide (strict)"("Value"=w282, "Scale.Minimum"=w284, "Scale.Maximum"=w283, "Scale.Increment"=w281) -> ()  [unwired: 2 in, 2 out]
            n161 = property on="On/Off" class="Bool (strict)"("Visible"=w286) -> ()  [unwired: 2 in, 2 out]
            n162 = property on="Test Slider" class="Slide (strict)"("Visible"=w286) -> ()  [unwired: 2 in, 2 out]
            n163 = property on="Test Ring" class="Ring (strict)"("Visible"=w286) -> ()  [unwired: 2 in, 2 out]
            n164 = property on="Rev/Fwd" class="Clust (strict)"("Visible"=w286) -> ()  [unwired: 2 in, 2 out]
          }
          frame "Servo" {
            w302 = FALSE ("Visible")
            n165 = call <vilib>:"NT Read Number.vi"("name"=w304) -> ("value"=w303:dbl)  [unwired: 8 in, 2 out]
            n166 = property on="Test Slider" class="Slide (strict)"("Visible"=TRUE, "Scale.Maximum"=170.0 ("Scale.Range:Maximum")) -> ()  [unwired: 2 in, 2 out]
            n167 = local write "Test Slider"(w303) -> ()
            n168 = property on="Motor" class="Clust (strict)"("Visible"=w302) -> ()  [unwired: 2 in, 2 out]
            n169 = property on="Rev/Fwd" class="Clust (strict)"("Visible"=w302) -> ()  [unwired: 2 in, 2 out]
            n170 = property on="On/Off" class="Bool (strict)"("Visible"=w302) -> ()  [unwired: 2 in, 2 out]
            n171 = property on="Test Ring" class="Ring (strict)"("Visible"=w302) -> ()  [unwired: 2 in, 2 out]
          }
          frame "Relay", "Solenoid" {
            w305 = FALSE ("Visible")
            n172 = property on="Motor" class="Clust (strict)"("Visible"=w305) -> ()  [unwired: 2 in, 2 out]
            n173 = property on="Test Slider" class="Slide (strict)"("Visible"=w305) -> ()  [unwired: 2 in, 2 out]
            n174 = Search and Replace String(input string=w306, search string="/Value  **", replace string="/Direction") -> (result string=w312:string)  [unwired: 5 in, 3 out]
            n175 = property on="Test Ring" class="Ring (strict)"("Visible"=w305) -> ()  [unwired: 2 in, 2 out]
            n176 = call <vilib>:"NT Read String.vi"("name"=w312) -> ("value"=w310:string)  [unwired: 8 in, 2 out]
            n177 = Equal?(x="Both directions", y=w310) -> (x = y?=w308:bool)
            n178 = Not(x=w308) -> (.not. x?=w309:bool)
            n179 = property on="Rev/Fwd" class="Clust (strict)"("Visible"=w308) -> ()  [unwired: 2 in, 2 out]
            n180 = property on="On/Off" class="Bool (strict)"("Visible"=w309, "Caption.Text"=w307) -> ()  [unwired: 2 in, 2 out]
          }
          frame "Compressor", "Digital Out" {
            w315 = FALSE ("Visible")
            # "Get direction and finish"
            n181 = property on="Motor" class="Clust (strict)"("Visible"=w315) -> ()  [unwired: 2 in, 2 out]
            n182 = property on="Test Slider" class="Slide (strict)"("Visible"=w315) -> ()  [unwired: 2 in, 2 out]
            n183 = property on="Test Ring" class="Ring (strict)"("Visible"=w315) -> ()  [unwired: 2 in, 2 out]
            n184 = property on="On/Off" class="Bool (strict)"("Visible"=TRUE, "Caption.Text"=w316) -> ()  [unwired: 2 in, 2 out]
            n185 = property on="Rev/Fwd" class="Clust (strict)"("Visible"=FALSE) -> ()  [unwired: 2 in, 2 out]
          }
          frame "Camera" {
            n186 = call <vilib>:"NT_Get Last Path Segment.vi"("String in"=w323) -> ("String out"=w324:string)  [unwired: 10 in]
            n187 = property on="On/Off" class="Bool (strict)"("Visible"=FALSE) -> ()  [unwired: 2 in, 2 out]
            n188 = property on="Motor" class="Clust (strict)"("Visible"=FALSE) -> ()  [unwired: 2 in, 2 out]
            n189 = property on="Rev/Fwd" class="Clust (strict)"("Visible"=FALSE) -> ()  [unwired: 2 in, 2 out]
            n190 = case shown="\"White Balance  **\"" w324 {
              tunnel: w323 -> [w330 w339 w348 w357 w366 _ w372]
              tunnel: w322 -> [w328 w336 w345 w354 w363 _ _]
              frame "Size  **" {
                n191 = Index Array(array=w328) -> (element=w327:cluster{string[]})  [unwired: 1 in]
                n192 = call <vilib>:"NT Read String.vi"("name"=w330) -> ("value"=w329:string)  [unwired: 8 in, 2 out]
                n193 = Unbundle(w327) -> (w325:string[])
                n194 = Match First String(2:w325, 3:w329) -> (0:w326:i32)  [unwired: 1 out]
                n195 = property on="Test Ring" class="Ring (strict)"("Value"=w326, "Strings []"=w325) -> ()  [unwired: 2 in, 2 out]
                n196 = property on="Test Ring" class="Ring (strict)"("Visible"=TRUE) -> ()  [unwired: 2 in, 2 out]
                n197 = property on="Test Slider" class="Slide (strict)"("Visible"=FALSE) -> ()  [unwired: 2 in, 2 out]
              }
              frame "White Balance  **" {
                n198 = Index Array(array=w336, index=1) -> (element=w337:cluster{string[]})
                n199 = call <vilib>:"NT Read String.vi"("name"=w339) -> ("value"=w338:string)  [unwired: 8 in, 2 out]
                n200 = Unbundle(w337) -> (w334:string[])
                n201 = Match First String(2:w334, 3:w338) -> (0:w333:i32)  [unwired: 1 out]
                n202 = property on="Test Ring" class="Ring (strict)"("Value"=w333, "Strings []"=w334) -> ()  [unwired: 2 in, 2 out]
                n203 = property on="Test Ring" class="Ring (strict)"("Visible"=TRUE) -> ()  [unwired: 2 in, 2 out]
                n204 = property on="Test Slider" class="Slide (strict)"("Visible"=FALSE) -> ()  [unwired: 2 in, 2 out]
              }
              frame "Exposure  **" {
                n205 = Index Array(array=w345, index=2) -> (element=w346:cluster{string[]})
                n206 = call <vilib>:"NT Read String.vi"("name"=w348) -> ("value"=w347:string)  [unwired: 8 in, 2 out]
                n207 = Unbundle(w346) -> (w342:string[])
                n208 = Match First String(2:w342, 3:w347) -> (0:w343:i32)  [unwired: 1 out]
                n209 = property on="Test Ring" class="Ring (strict)"("Value"=w343, "Strings []"=w342) -> ()  [unwired: 2 in, 2 out]
                n210 = property on="Test Ring" class="Ring (strict)"("Visible"=TRUE) -> ()  [unwired: 2 in, 2 out]
                n211 = property on="Test Slider" class="Slide (strict)"("Visible"=FALSE) -> ()  [unwired: 2 in, 2 out]
              }
              frame "Exposure Priority  **" {
                n212 = Index Array(array=w354, index=3) -> (element=w355:cluster{string[]})
                n213 = call <vilib>:"NT Read String.vi"("name"=w357) -> ("value"=w356:string)  [unwired: 8 in, 2 out]
                n214 = Unbundle(w355) -> (w351:string[])
                n215 = Match First String(2:w351, 3:w356) -> (0:w352:i32)  [unwired: 1 out]
                n216 = property on="Test Ring" class="Ring (strict)"("Value"=w352, "Strings []"=w351) -> ()  [unwired: 2 in, 2 out]
                n217 = property on="Test Ring" class="Ring (strict)"("Visible"=TRUE) -> ()  [unwired: 2 in, 2 out]
                n218 = property on="Test Slider" class="Slide (strict)"("Visible"=FALSE) -> ()  [unwired: 2 in, 2 out]
              }
              frame "Color Enable  **" {
                n219 = Index Array(array=w363, index=4) -> (element=w364:cluster{string[]})
                n220 = call <vilib>:"NT Read String.vi"("name"=w366) -> ("value"=w365:string)  [unwired: 8 in, 2 out]
                n221 = Unbundle(w364) -> (w360:string[])
                n222 = Match First String(2:w360, 3:w365) -> (0:w361:i32)  [unwired: 1 out]
                n223 = property on="Test Ring" class="Ring (strict)"("Value"=w361, "Strings []"=w360) -> ()  [unwired: 2 in, 2 out]
                n224 = property on="Test Ring" class="Ring (strict)"("Visible"=TRUE) -> ()  [unwired: 2 in, 2 out]
                n225 = property on="Test Slider" class="Slide (strict)"("Visible"=FALSE) -> ()  [unwired: 2 in, 2 out]
              }
              frame Default {
                n226 = property on="Test Ring" class="Ring (strict)"("Visible"=FALSE) -> ()  [unwired: 2 in, 2 out]
                n227 = property on="Test Slider" class="Slide (strict)"("Visible"=FALSE) -> ()  [unwired: 2 in, 2 out]
              }
              frame "Brightness  **", "Color Level  **", "Compression  **", "FPS  **", "Sharpness  **" {
                n228 = call <vilib>:"NT Read Number.vi"("name"=w372) -> ("value"=w371:dbl)  [unwired: 8 in, 2 out]
                n229 = local write "Test Slider"(w371) -> ()
                n230 = property on="Test Ring" class="Ring (strict)"("Visible"=FALSE) -> ()  [unwired: 2 in, 2 out]
                n231 = property on="Test Slider" class="Slide (strict)"("Visible"=TRUE, "Scale.Maximum"=100.0 ("Scale.Range:Maximum")) -> ()  [unwired: 2 in, 2 out]
              }
            }
          }
        }
        n232 = property on="Progress" class="Clust (strict)"("Visible"=FALSE) -> ()  [unwired: 2 in, 2 out]
      }
      event "Test Name": Mouse Enter {
        # "Populate the ring with the list of tests"
        n233 = event-data() -> ()  [unwired: 1 in, 1 out]
        n234 = call <vilib>:"NT Read String Array.vi"("name"="TestMode/TestList" ("Name")) -> ("value"=w379:string[])  [unwired: 8 in, 2 out]
        n235 = Build Array (concatenate)("Select the test to run...", w379) -> (w378:string[])
        n236 = property on="Test Name" class="Ring (strict)"("Strings []"=w378) -> ()  [unwired: 2 in, 2 out]
      }
      event "Test Name": Value Change {
        w380 = FALSE ("Visible")
        # "Tell the robot the test name to run"
        n237 = event-data() -> ("NewVal"=w384:u16)  [unwired: 1 in]
        n238 = property on="Test Name" class="Ring (strict)"() -> ("Strings []"=w385:string[])  [unwired: 2 in, 2 out]
        n239 = local write "Progress"(T8 {"Test Progress"=0, "Test Progress Text"=""} ("Progress")) -> ()
        n240 = Index Array(array=w385, index=w384) -> (element=w383:string)
        n241 = call <vilib>:"NT Write String.vi"("value"=w383, "name"="TestMode/TestName" ("Name")) -> ()  [unwired: 9 in, 1 out]
        n242 = property on="Progress" class="Clust (strict)"("Visible"=TRUE) -> ()  [unwired: 2 in, 2 out]
        n243 = property on="Motor" class="Clust (strict)"("Visible"=w380) -> ()  [unwired: 2 in, 2 out]
        n244 = property on="Test Slider" class="Slide (strict)"("Visible"=w380) -> ()  [unwired: 2 in, 2 out]
        n245 = property on="On/Off" class="Bool (strict)"("Visible"=w380) -> ()  [unwired: 2 in, 2 out]
        n246 = property on="Rev/Fwd" class="Clust (strict)"("Visible"=w380) -> ()  [unwired: 2 in, 2 out]
        n247 = property on="Test Ring" class="Ring (strict)"("Visible"=w380) -> ()  [unwired: 2 in, 2 out]
      }
      event "Select Auto": Mouse Enter {
        # "Populate the combo box with the list of autonomous options"
        n248 = event-data() -> ()  [unwired: 1 in, 1 out]
        n249 = call <vilib>:"NT Read String Array.vi"("name"="Auto List" ("Name")) -> ("value"=w387:string[])  [unwired: 8 in, 2 out]
        n250 = property on="Select Auto" class="CmbBox"("Strings[]"=w387) -> ()  [unwired: 2 in, 2 out]
      }
      event "Select Auto": Value Change {
        # "User modified the Auto Selection. Write to NT variable so robot knows."
        n251 = event-data() -> ("NewVal"=w389:string)  [unwired: 1 in]
        n252 = call <vilib>:"NT Write String.vi"("value"=w389, "name"="Auto Selector" ("Name")) -> ()  [unwired: 9 in, 1 out]
      }
      event "CheckList": Double Click {
        # "Shift clears all"
        # "Update symbols on the listbox"
        n253 = event-data() -> ("PlatMods.Shift"=w391:bool, "Row"=w393:i32)  [unwired: 1 in]
        n254 = case shown="True" w391 {
          tunnel: w393 -> [w397 _]
          tunnel: 1 -> [w396 _]
          frame False {
            n255 = property on="CheckList" class="LstBox (strict)"() -> ("Item Symbols"=w395:i32[])  [unwired: 2 in, 2 out]
            n256 = Replace Array Subset(array=w395, new element=w396, index=w397) -> (w394:i32[])
            n257 = property on="CheckList" class="LstBox (strict)"("Item Symbols"=w394) -> ()  [unwired: 2 in, 2 out]
          }
          frame True {
            w398 = 0 ("Top Row")
            n258 = property on="CheckList" class="LstBox (strict)"() -> ("Number of Rows"=w400:u32)  [unwired: 2 in, 2 out]
            n259 = Initialize Array(0, w400) -> (w399:i32[])
            n260 = property on="CheckList" class="LstBox (strict)"("Top Row"=w398, "Value"=w398, "Item Symbols"=w399) -> ()  [unwired: 2 in, 2 out]
          }
        }
      }
      event "CheckList": Key Down {
        # "Update symbols on the listbox\nLeft and right keys check and uncheck"
        n261 = event-data() -> ("VKey"=w403:T24)  [unwired: 1 in]
        n262 = case shown="\"Left\", \"Right\"" w403 {
          selector: w403 -> [w408 _]
          tunnel: eventvkey."Left" ("VKey") -> [w406 _]
          frame "Left", "Right" {
            n263 = Equal?(x=w406, y=w408) -> (x = y?=w407:bool)
            n264 = Select(t=0, s=w407, f=1) -> (s? t:f=w409:i32)
            n265 = property on="CheckList" class="LstBox (strict)"() -> ("Item Symbols"=w412:i32[])  [unwired: 2 in, 2 out]
            n266 = Replace Array Subset(array=w412, new element=w409, index="CheckList") -> (w411:i32[])
            n267 = property on="CheckList" class="LstBox (strict)"("Item Symbols"=w411) -> ()  [unwired: 2 in, 2 out]
          }
          frame Default {
          }
        }
      }
      event "Motor.Enable": Value Change {
        # "When the test mode otor enable helper is set, update that\ntree row item's value"
        n268 = event-data() -> ("NewVal"=w417:bool)  [unwired: 1 in]
        n269 = Unbundle("Motor") -> ("Value"=w416:dbl)  [unwired: 1 out]
        n270 = Select(t=w416, s=w417, f=0.0) -> (s? t:f=w414:dbl)
        n271 = call <vilib>:"NT Write Number.vi"("value"=w414, "name"=w413) -> ()  [unwired: 9 in, 1 out]
      }
      event "Test Slider": Value Change {
        # "When the test mode slider helper is set, update that\ntree row item's value"
        n272 = event-data() -> ("NewVal"=w419:dbl)  [unwired: 1 in]
        n273 = call <vilib>:"NT Write Number.vi"("value"=w419, "name"=w420) -> ()  [unwired: 9 in, 1 out]
      }
      event "On/Off": Value Change {
        # "When the test mode on/off helper value is set, update that\ntree row item's value"
        n274 = event-data() -> ("NewVal"=w423:bool)  [unwired: 1 in]
        n275 = Boolean To (0,1)(Boolean=w423) -> (0, 1=w422:i16)
        n276 = call <vilib>:"NT Write Number.vi"("value"=w422, "name"=w421) -> ()  [unwired: 9 in, 1 out]
      }
      event "Rev/Fwd": Value Change {
        # "When the test mode helper value for relays is set, update that\ntree row item's value"
        n277 = event-data() -> ("NewVal.Forward"=w430:bool, "NewVal.Reverse"=w429:bool)  [unwired: 1 in]
        n278 = Boolean To (0,1)(Boolean=w430) -> (0, 1=w426:i16)
        n279 = Boolean To (0,1)(Boolean=w429) -> (0, 1=w428:i16)
        n280 = Negate(x=w428) -> (-x=w427:i16)
        n281 = Add(x=w426, y=w427) -> (x+y=w425:i16)
        n282 = call <vilib>:"NT Write Number.vi"("value"=w425, "name"=w424) -> ()  [unwired: 9 in, 1 out]
      }
      event "Test Ring": Value Change {
        # "When a test mode helper value is selected from the ring,\nset the tree item's variable to the string value"
        n283 = event-data() -> ("NewVal"=w433:u16)  [unwired: 1 in]
        n284 = property on="Test Ring" class="Ring (strict)"() -> ("Strings []"=w434:string[])  [unwired: 2 in, 2 out]
        n285 = Index Array(array=w434, index=w433) -> (element=w432:string)
        n286 = call <vilib>:"NT Write String.vi"("value"=w432, "name"=w431) -> ()  [unwired: 9 in, 1 out]
      }
      event "Rec Mode": Value Change {
        # "Update globals for recording mode and path to read log from.\nClear when logging and let NetworkTables set path for vision to\nuse."
        n287 = event-data() -> ("NewVal"=w443:enum32{"Stop", "Record", "Playback"})  [unwired: 1 in]
        n288 = global write "WPI_DashboardLogging Global.vi" "Logging Filename"(path "") -> ()
        n289 = global write "WPI_DashboardLogging Global.vi" "Recording"(w443) -> ()
        n290 = case shown="\"Playback\"" w443 {
          tunnel: w442 -> [_ w445 w453]
          tunnel: [_ _ w452] -> w440
          tunnel: [_ _ w451] -> _
          tunnel: w438 -> [_ _ w449]
          tunnel: cluster{i32, i32} {-250, 170} -> [_ _ w448]
          tunnel: [_ _ T25 {"Image Size"=TRUE, "Image Type"=TRUE, "Pixel Value"=TRUE, "ROI Information"=TRUE, "Zoom Factor"=FALSE} ("Image Information Shown:All Elements")] -> w435
          tunnel: [_ _ TRUE ("Zoom Factor")] -> w436
          frame Default {
          }
          frame "Stop", "Record" {
            # "Place Window too"
            n291 = invoke class="VI" method="FP.Close"(reference=w445) -> (reference out=w444:refnum<vi>)  [unwired: 2 in, 2 out]
            n292 = invoke class="VI" method="Abort VI"(reference=w444) -> ()  [unwired: 2 in, 3 out]
          }
          frame "Playback" {
            n293 = call "Open Playback Panel.vi"("Offset"=w448, "DB VI Ref"=w449, "Playback in"=w453) -> ("Playback out"=w450:refnum<vi>)  [unwired: 8 in]
            n294 = register-events(w450) -> (reference out=w452:refnum<event-registration>, error out=w451:errorcluster)  [unwired: 2 in]
          }
        }
        n295 = property on="Camera Image Right" class="ImageControl"("Image Information Shown"=w435, "Image Information Visible"=w436) -> ()  [unwired: 2 in, 2 out]
        n296 = property on="Camera Image" class="ImageControl"("Image Information Shown"=w435, "Image Information Visible"=w436) -> ()  [unwired: 2 in, 2 out]
        n297 = call <vilib>:"WPI_DashboardNT Log FieldName Cache.vi"("Operation"=enum16{"Lookup/Add", "Index", "Clear"}."Clear") -> ()  [unwired: 8 in, 3 out]
      }
      event Panel Close {
        w454 = enum32{"Stop", "Record", "Playback"}."Stop" ("Rec Mode")
        # "Playback window has been closed, abort"
        n298 = event-data() -> ()  [unwired: 1 in, 4 out]
        n299 = local write "Rec Mode"(w454) -> ()
        n300 = global write "WPI_DashboardLogging Global.vi" "Recording"(w454) -> ()
      }
      event Panel Close {
        # "Abort playback window and ourself"
        n301 = event-data() -> ()  [unwired: 1 in, 4 out]
        n302 = invoke class="VI" method="FP.Close"(reference=w457) -> (reference out=w456:refnum<vi>)  [unwired: 2 in, 2 out]
        n303 = invoke class="VI" method="Abort VI"(reference=w456) -> (error out=w455:errorcluster)  [unwired: 2 in, 2 out]
        n304 = invoke class="VI" method="Abort VI"(error in=w455) -> ()  [unwired: 2 in, 3 out]
      }
      event "Tree": Double Click {
        n305 = event-data() -> ("PlatMods"=w463:T27, "Tag"=w460:string)  [unwired: 1 in]
        n306 = Unbundle(w463) -> ("Shift"=w462:bool)  [unwired: 4 out]
        n307 = String Subset(string=w460, length (rest)=1 ("length (rest)")) -> (substring=w459:string)  [unwired: 1 in]
        n308 = Not(x=w462) -> (.not. x?=w461:bool)
        n309 = case shown="\"/\"" w459 {
          tunnel: w460 -> [_ w465]
          tunnel: w461 -> [_ w464]
          frame Default {
          }
          frame "/" {
            n310 = call <vilib>:"NT Update Persistence.vi"("Persistence"=w464, "Name"=w465) -> ()  [unwired: 9 in, 1 out]
          }
        }
      }
    }
  }
  n311 = while {
    tunnel: w54 -> [w467]
    i -> [w470]
    stop <- FALSE stop-if-true
    n312 = Wait (ms)(milliseconds to wait=u32 100) -> ()  [unwired: 1 out]
    n313 = case shown="\"Playback\"" "Rec Mode" {
      tunnel: w470 -> [_ _ w485]
      tunnel: [u32 2829099 ("Base Color") u32 11141120 ("Target Color") w474] -> w466
      frame "Stop", Default {
        # "Reset the color, extra updates don't cost much"
      }
      frame "Record" {
      }
      frame "Playback" {
        # "Playback"
        n314 = Quotient & Remainder(x=w485, y=u32 50 ("milliseconds to wait")) -> (x-y*floor(x/y)=w481:u32)  [unwired: 1 out]
        n315 = Divide(x=w481, y=u32 50 ("milliseconds to wait")) -> (x/y=w478:dbl)
        n316 = Multiply(x=6.283185307179586, y=w478) -> (x*y=w483:dbl)
        n317 = Sine(x=w483) -> (sin(x)=w482:dbl)
        n318 = Absolute Value(x=w482) -> (abs(x)=w475:dbl)
        n319 = call "Interpolate RGB Color.vi"("Proportion"=w475, "Target Color"=u32 30976, "Base Color"=u32 2829099) -> ("Result Color"=w474:u32)  [unwired: 8 in]
      }
    }
    n320 = property class="Pane"(reference=w467, "PaneColor"=w466) -> ()  [unwired: 1 in, 2 out]
  }
  n321 = local write "Dashboard Tab"(T2."Arm 2" ("Dashboard Tab")) -> ()
  n322 = property on="On/Off" class="Bool (strict)"("Visible"=w26) -> ()  [unwired: 2 in, 2 out]
  n323 = property on="Motor" class="Clust (strict)"("Visible"=w26) -> ()  [unwired: 2 in, 2 out]
  n324 = property on="Progress" class="Clust (strict)"("Visible"=w26) -> ()  [unwired: 2 in, 2 out]
  n325 = property on="Test Ring" class="Ring (strict)"("Visible"=w26) -> ()  [unwired: 2 in, 2 out]
  n326 = property on="Rev/Fwd" class="Clust (strict)"("Visible"=w26) -> ()  [unwired: 2 in, 2 out]
  n327 = while {
    tunnel: u16 1741 ("timeout ms (25000)") -> [w487]
    stop <- FALSE stop-if-true
    n328 = TCP Create Listener(10:w487) -> (0:w486:errorcluster, 3:w488:refnum<k5>)  [unwired: 4 in, 1 out]
    n329 = case shown="No Error" w486 {
      selector: w486 -> [w490 _]
      tunnel: w488 -> [w491 _]
      frame No Error {
        n330 = while {
          tunnel: w491 -> [w494]
          tunnel: w490 -> [w493]
          stop <- FALSE stop-if-true
          n331 = TCP Wait On Listener(8:w493, 11:w494) -> (0:w495:errorcluster, 4:w496:refnum<k5>)  [unwired: 2 in, 3 out]
          n332 = local write "TCP"(w496) -> ()
          n333 = case shown="Error" w495 {
            frame No Error {
            }
            frame Error {
              n334 = Wait (ms)(milliseconds to wait=u32 1000) -> ()  [unwired: 1 out]
            }
          }
        }
      }
      frame Error {
        n335 = Wait (ms)(milliseconds to wait=u32 1000) -> ()  [unwired: 1 out]
      }
    }
  }
  n336 = global write "WPI_DashboardLogging Global.vi" "Recording"(w49) -> ()
  n337 = local write "Rec Mode"(w49) -> ()
  n338 = call <vilib>:"NT Write String.vi"("value"="Select Auto", "name"="Auto Selector" ("Name")) -> ()  [unwired: 9 in, 1 out]
